vi "1.3.6-Transform.vi"(9 "Lidar Vertical Position":i8, 10 "Lidar Distance":u16, 11 "Lidar Scan Angle":u8) -> (0 "Is object?":bool, 1 "Robot Z":i16, 2 "Robot Y":i16, 3 "Lidar X = Robot X":i16, 4 "Distance Object":i16, 5 "object distance squared":i16)   [LabVIEW 2010]
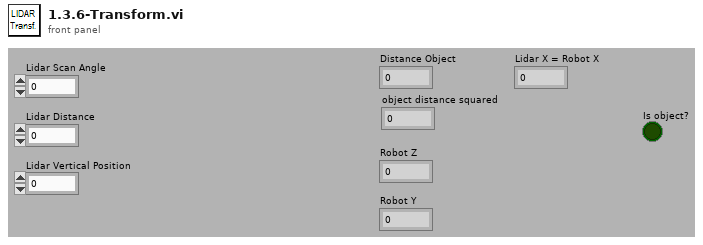
[diagram p1: front panel]
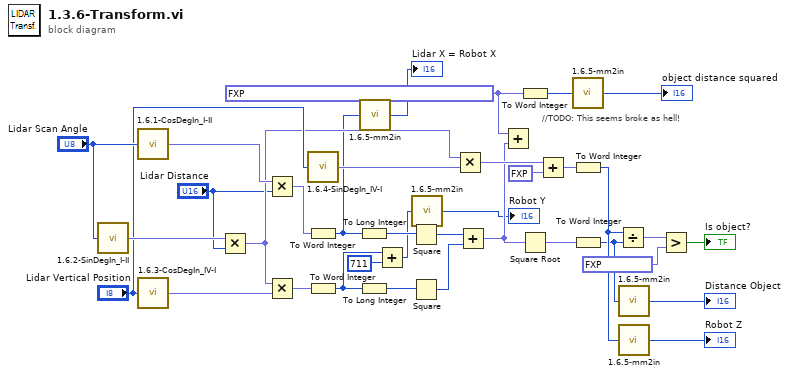
[diagram p0: block diagram]
diagram:
  w10 = fxp<+,64,32> 0.0 ("x")
  # "//TODO: This seems broke as hell!"
  n1 = call "1.6.2-SinDegIn_I-II.vi"("theta"="Lidar Scan Angle") -> ("Numeric"=w29:fxp<+/-,16,1>)
  n2 = call "1.6.1-CosDegIn_I-II.vi"("theta"="Lidar Scan Angle") -> ("Numeric"=w30:fxp<+/-,16,1>)
  n3 = call "1.6.3-CosDegIn_IV-I.vi"("theta"="Lidar Vertical Position") -> ("Numeric"=w27:fxp<+/-,16,1>)
  n4 = Multiply(x=w29, y="Lidar Distance") -> (x*y=w21:fxp<+/-,32,16>)
  n5 = Multiply(x=w30, y="Lidar Distance") -> (x*y=w22:fxp<+/-,16,16>)
  n6 = Multiply(x=w21, y=w27) -> (x*y=w20:fxp<+/-,16,16>)
  n7 = call "1.6.4-SinDegIn_IV-I.vi"("theta"="Lidar Vertical Position") -> ("Numeric"=w26:fxp<+/-,16,1>)
  n8 = To Word Integer(number=w22) -> (16bit integer=w12:i16)
  n9 = To Word Integer(number=w20) -> (16bit integer=w1:i16)
  n10 = To Long Integer(number=w12) -> (32bit integer=w16:i32)
  n11 = To Long Integer(number=w1) -> (32bit integer=w15:i32)
  n12 = call "1.6.5-mm2in.vi"("mm"=w12) -> ("in"=→"Lidar X = Robot X":i16)
  n13 = Add(x=w1, y=i16 711) -> (x+y=w2:i16)
  n14 = Square(x=w16) -> (x^2=w34:i32)
  n15 = Square(x=w15) -> (x^2=w35:i32)
  n16 = call "1.6.5-mm2in.vi"("mm"=w2) -> ("in"=→"Robot Y":i16)
  n17 = Multiply(x=w21, y=w26) -> (x*y=w24:fxp<+/-,18,18>)
  n18 = Add(x=w34, y=w35) -> (x+y=w11:fxp<+,64,32>)
  n19 = Add(x=w10, y=w11) -> ()  [unwired: 1 out]
  n20 = To Word Integer(number=w10) -> (16bit integer=w4:i16)
  n21 = Square Root(x=w11) -> (sqrt(x)=w18:fxp<+/-,16,16>)
  n22 = Add(x=w24, y=fxp<+/-,18,18> 692.0) -> (x+y=w19:fxp<+/-,16,16>)
  n23 = call "1.6.5-mm2in.vi"("mm"=w4) -> ("in"=→"object distance squared":i16)
  n24 = To Word Integer(number=w19) -> (16bit integer=w8:i16)
  n25 = To Word Integer(number=w18) -> (16bit integer=w6:i16)
  n26 = Divide(x=w8, y=w6) -> (x/y=w33:fxp<+/-,32,16>)
  n27 = call "1.6.5-mm2in.vi"("mm"=w6) -> ("in"=→"Distance Object":i16)
  n28 = call "1.6.5-mm2in.vi"("mm"=w8) -> ("in"=→"Robot Z":i16)
  n29 = Greater?(x=w33, y=fxp<+,8,-2> 0.150390625) -> (0:→"Is object?":bool)
